vi "MessageName.vi"() -> (2 "MessageName":string)   [LabVIEW 2020, in "Empty.lvlib"]
uses:
  Empty.lvlib
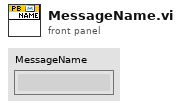
[diagram p1: front panel]
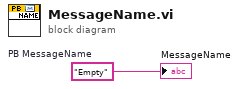
[diagram p0: block diagram]
diagram:
  w1 = "Empty"  # PB MessageName
  "MessageName" <- w1
